vi "_Worker Drop Instance FG.vi"(11 "Worker Path In":path) -> (3 "Worker Path":path)   [LabVIEW 2022 SP3, in "FlexBlocks Support.lvlib"]
uses:
  FlexBlocks Support.lvlib
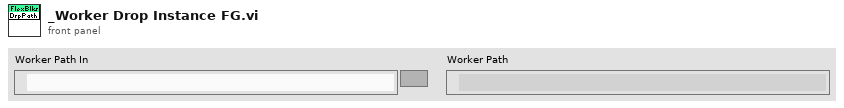
[diagram p1: front panel]
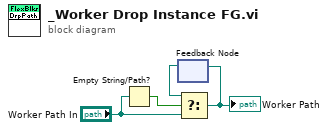
[diagram p0: block diagram]
diagram:
  n1 = Empty String/Path?(string/path="Worker Path In") -> (empty?=w1:bool)
  n2 = feedback #1() -> (w3:path)  [unwired: 1 in]
  n3 = Select(t=w3, s=w1, f="Worker Path In") -> (s? t:f=w4:path)
  "Worker Path" <- w4
  n4 = feedback-in #1(w4) -> ()
